vi "MFC Flow.vi"(8 "error in (no error)":errorcluster, 10 "MFC Flow":waveform(dbl), 11 "Mass Flow Controllers in":refnum<class "Mass Flow Controllers.lvclass">) -> (0 "error out":errorcluster, 3 "Mass Flow Controllers out":refnum<class "Mass Flow Controllers.lvclass">)   [LabVIEW 2021, in "Mass Flow Controllers.lvclass"]
uses:
  Mass Flow Controllers.lvclass
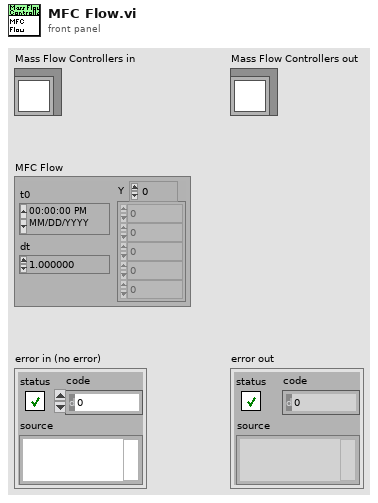
[diagram p1: front panel]
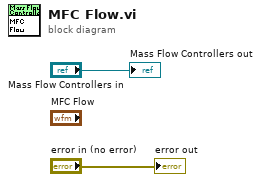
[diagram p0: block diagram]
diagram:
  "error out" <- "error in (no error)"
  "Mass Flow Controllers out" <- "Mass Flow Controllers in"
